vi "HTTP GET JSON Current Time.vi"() -> ()   [LabVIEW 2020, in "HTTP GET Current Time.lvlib"]
uses:
  rest_api_time_cluster.ctl
  HTTP GET Current Time.lvlib
  <vilib>/httpClient/LabVIEWHTTPClient.lvlib
  JKI JSON Serialization.lvlib
panel:
  out "raw json response":string
  in  "url":string="http://worldclockapi.com/api/json/utc/now"
  out "error out":errorcluster
  out "time":T1
  in  "error in":errorcluster
  # "This example get's the current UTC time"
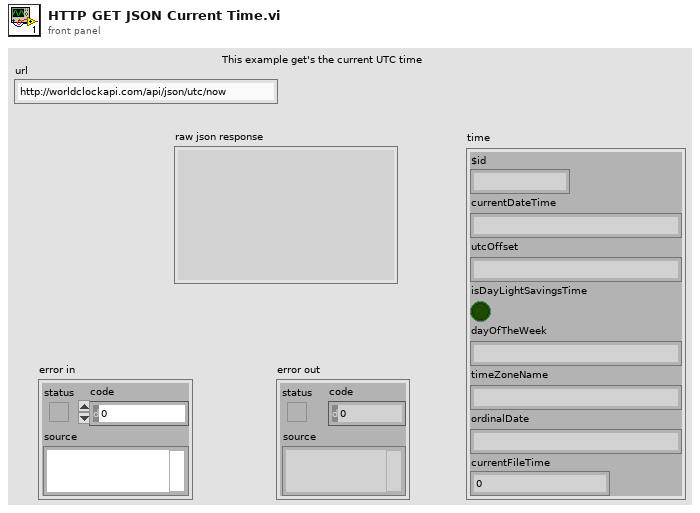
[diagram p1: front panel]
types:
  T1 = typedef "HTTP GET Current Time.lvlib/rest_api_time_cluster.ctl" = cluster{"$id":string, "currentDateTime":string, "utcOffset":string, "isDayLightSavingsTime":bool, "dayOfTheWeek":string, "timeZoneName":string, "ordinalDate":string, "currentFileTime":u64}
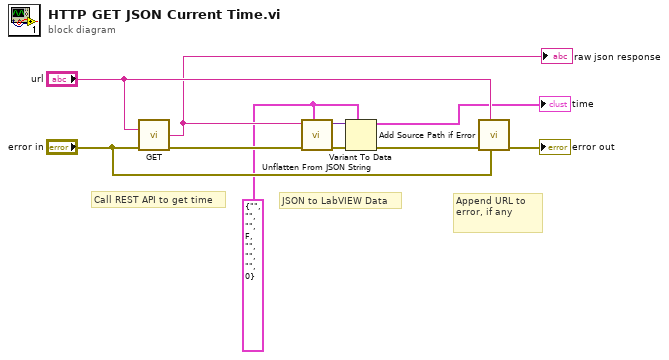
[diagram p0: block diagram]
diagram:
  w1 = T1 {"$id"="", "currentDateTime"="", "utcOffset"="", "isDayLightSavingsTime"=FALSE, "dayOfTheWeek"="", "timeZoneName"="", "ordinalDate"="", "currentFileTime"=0} ("time")
  # "JSON to LabVIEW Data"
  # "Call REST API to get time"
  # "Append URL to error, if any"
  n1 = call <vilib>:"GET.vi"("url"="url", "error in (no error)"="error in") -> ("body"=w7:string, "error out"=w2:errorcluster)  [unwired: 10 in, 2 out]
  "raw json response" <- w7
  n2 = call "Unflatten From JSON String.vi"("Type and Defaults"=w1, "error in"=w2, "JSON String"=w7) -> ("error out"=w9:errorcluster, "Variant"=w4:variant)  [unwired: 7 in]
  n3 = Variant To Data(error in=w9, type=w1, Variant=w4) -> (data=→"time":T1, error out=w5:errorcluster)
  n4 = call "Add Source Path if Error.vi"("Upstream Error"="error in", "Source Path or URL"="url", "error in"=w5) -> ("error out"=→"error out":errorcluster)  [unwired: 8 in]
